vi "Notifier_Driver.vi"(0 "Notification":bool, 2 "Notifier_Name":string, 11 "Error_In":errorcluster, 13 "Notifier_Operation_Select":T1=enum."Release_Notifier") -> (4 "Latest_Notification":bool, 15 "Error_Out":errorcluster)   [LabVIEW 2023]
doc: "Used to send the notification from one loop to other"
uses:
  Controls/Notifier_Operation_Select.ctl
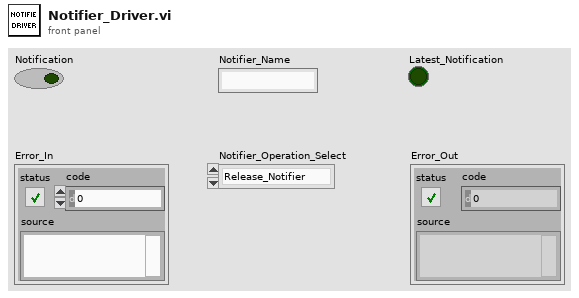
[diagram p1: front panel]
types:
  T1 = typedef "Notifier_Operation_Select.ctl" = enum16{"Obtain_Notifier", "Send_Notification", "Get_Notifier_Status", "Release_Notifier"}
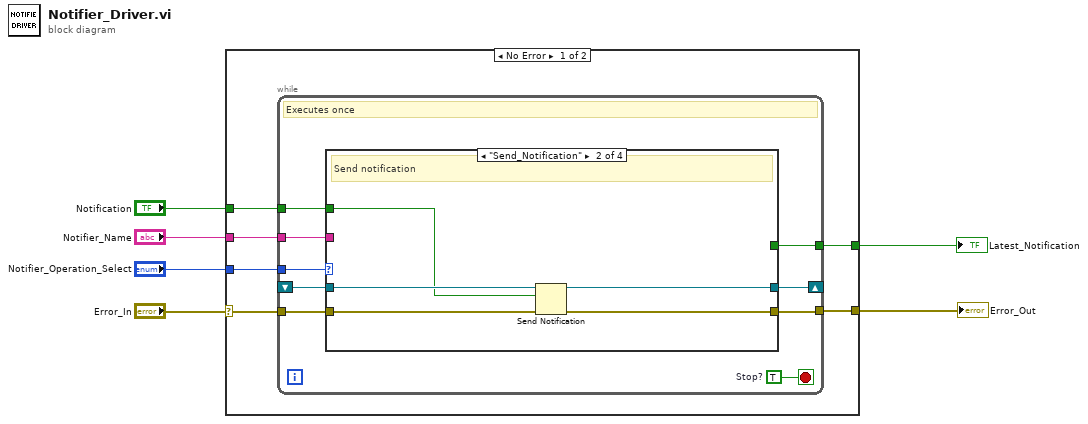
[diagram p0: block diagram]
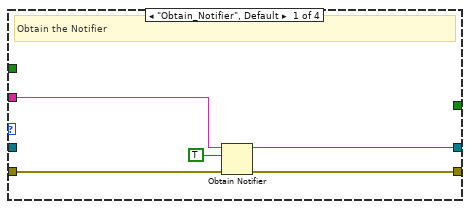
[diagram p2: hidden frame]
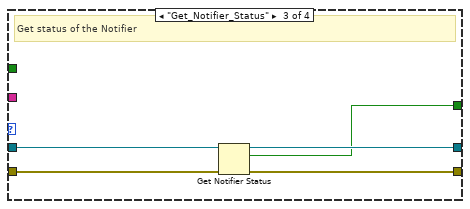
[diagram p3: hidden frame]
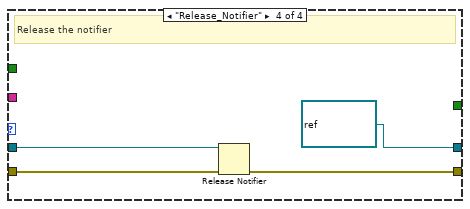
[diagram p4: hidden frame]
diagram:
  n1 = case shown="No Error" "Error_In" {
    selector: "Error_In" -> [w7 w41]
    tunnel: [w12 w41] -> w6
    tunnel: "Notifier_Operation_Select" -> [w11 _]
    tunnel: "Notifier_Name" -> [w10 _]
    tunnel: [w9 _] -> w3
    tunnel: "Notification" -> [w8 _]
    frame No Error {
      n2 = while {
        tunnel: w7 -> [w13]
        tunnel: [w21] -> w12
        tunnel: w11 -> [w20]
        shift-right: [w18] -> _
        shift-left: _ -> [w19]
        tunnel: w10 -> [w17]
        tunnel: [w15] -> w9
        tunnel: w8 -> [w14]
        stop <- w16 stop-if-true
        w16 = TRUE  # Stop?
        # "Executes once"
        n3 = case shown="\"Send_Notification\"" w20 {
          tunnel: w13 -> [w26 w31 w36 w40]
          tunnel: [w25 w30 w35 w39] -> w21
          tunnel: w19 -> [_ w29 w33 w38]
          tunnel: [w24 w28 w34 refnum<notifier> refnum ("notifier out")] -> w18
          tunnel: w17 -> [w22 _ _ _]
          tunnel: [_ _ w32 _] -> w15
          tunnel: w14 -> [_ w27 _ _]
          frame "Obtain_Notifier", Default {
            # "Obtain the Notifier"
            n4 = Obtain Notifier(name (unnamed)=w22, notification data type=TRUE, error in (no error)=w26) -> (notifier out=w24:refnum<notifier>, error out=w25:errorcluster)  [unwired: 1 in, 1 out]
          }
          frame "Send_Notification" {
            # "Send notification"
            n5 = Send Notification(notification=w27, notifier=w29, error in (no error)=w31) -> (notifier out=w28:refnum<notifier>, error out=w30:errorcluster)
          }
          frame "Get_Notifier_Status" {
            # "Get status of the Notifier"
            n6 = Get Notifier Status(notifier=w33, error in (no error)=w36) -> (notifier out=w34:refnum<notifier>, current notification=w32:bool, error out=w35:errorcluster)  [unwired: 2 out]
          }
          frame "Release_Notifier" {
            # "Release the notifier"
            n7 = Release Notifier(notifier=w38, error in (no error)=w40) -> (error out=w39:errorcluster)  [unwired: 1 in, 2 out]
          }
        }
      }
    }
    frame Error {
    }
  }
  "Error_Out" <- w6
  "Latest_Notification" <- w3
